vi "USRP oneTx one Rx.vi"() -> ()   [LabVIEW 2021]
uses:
  <vilib>/addons/Modulation/Analog/controls/Complex Data Waveform.ctl
  <vilib>/measure/maspectr.llb/Power Spectrum and PSD Export Mode.ctl
  system stop.vi
  <vilib>/measure/matone.llb/Extract Single Tone Information 1 Chan (CDB).vi
  <vilib>/measure/maspectr.llb/FFT Power Spectrum and PSD for 1 Chan (CDB).vi
  <instrlib>/niUSRP/niUSRP Fetch Rx Data (CDB Cluster).vi
  <instrlib>/niUSRP/niUSRP Write Tx Data (CDB Cluster).vi
  <vilib>/addons/Modulation/niAMT.lvlib
  <vilib>/measure/NI_MAPro.lvlib
  <vilib>/Analysis/NI_AALPro.lvlib
panel:
  in  "Tab Control":T1(tab)
  in  "IQ rate Tx":dbl=100000.0 format="%#_6p"
  in  "carrier frequency Tx":dbl=100000.0 format="%#_6p"
  in  "Tx Gain":dbl format="%#_6f"
  in  "Tx IP":refnum<k15>
  out "coerced IQ rate Tx":dbl=100000.0 format="%#_6p"
  out "coerced carrier frequency Tx":dbl=100000.0 format="%#_6p"
  in  "Rx IP":refnum<k15>
  in  "Rx gain":dbl format="%#_6f"
  in  "Frequency":dbl format="%#_13g"
  in  "Duration":dbl format="%#_13g"
  out "coerced IQ rate Rx":dbl=100000.0 format="%#_6p"
  out "coerced carrier frequency Rx":dbl=100000.0 format="%#_6p"
  in  "number of samples":i64=100000
  out "Waveform Graph":dbl[](graph)
  out "Received Waveform Graph":cluster{"f0":dbl, "df":dbl, "magnitude":dbl[]}(graph)
  out "detected frequency":dbl format="%.2p"
  out "detected Amplitude":dbl format="%.2p"
  out "Threshold indices":i32[](array[numeric])
  out "Threshold count":i32
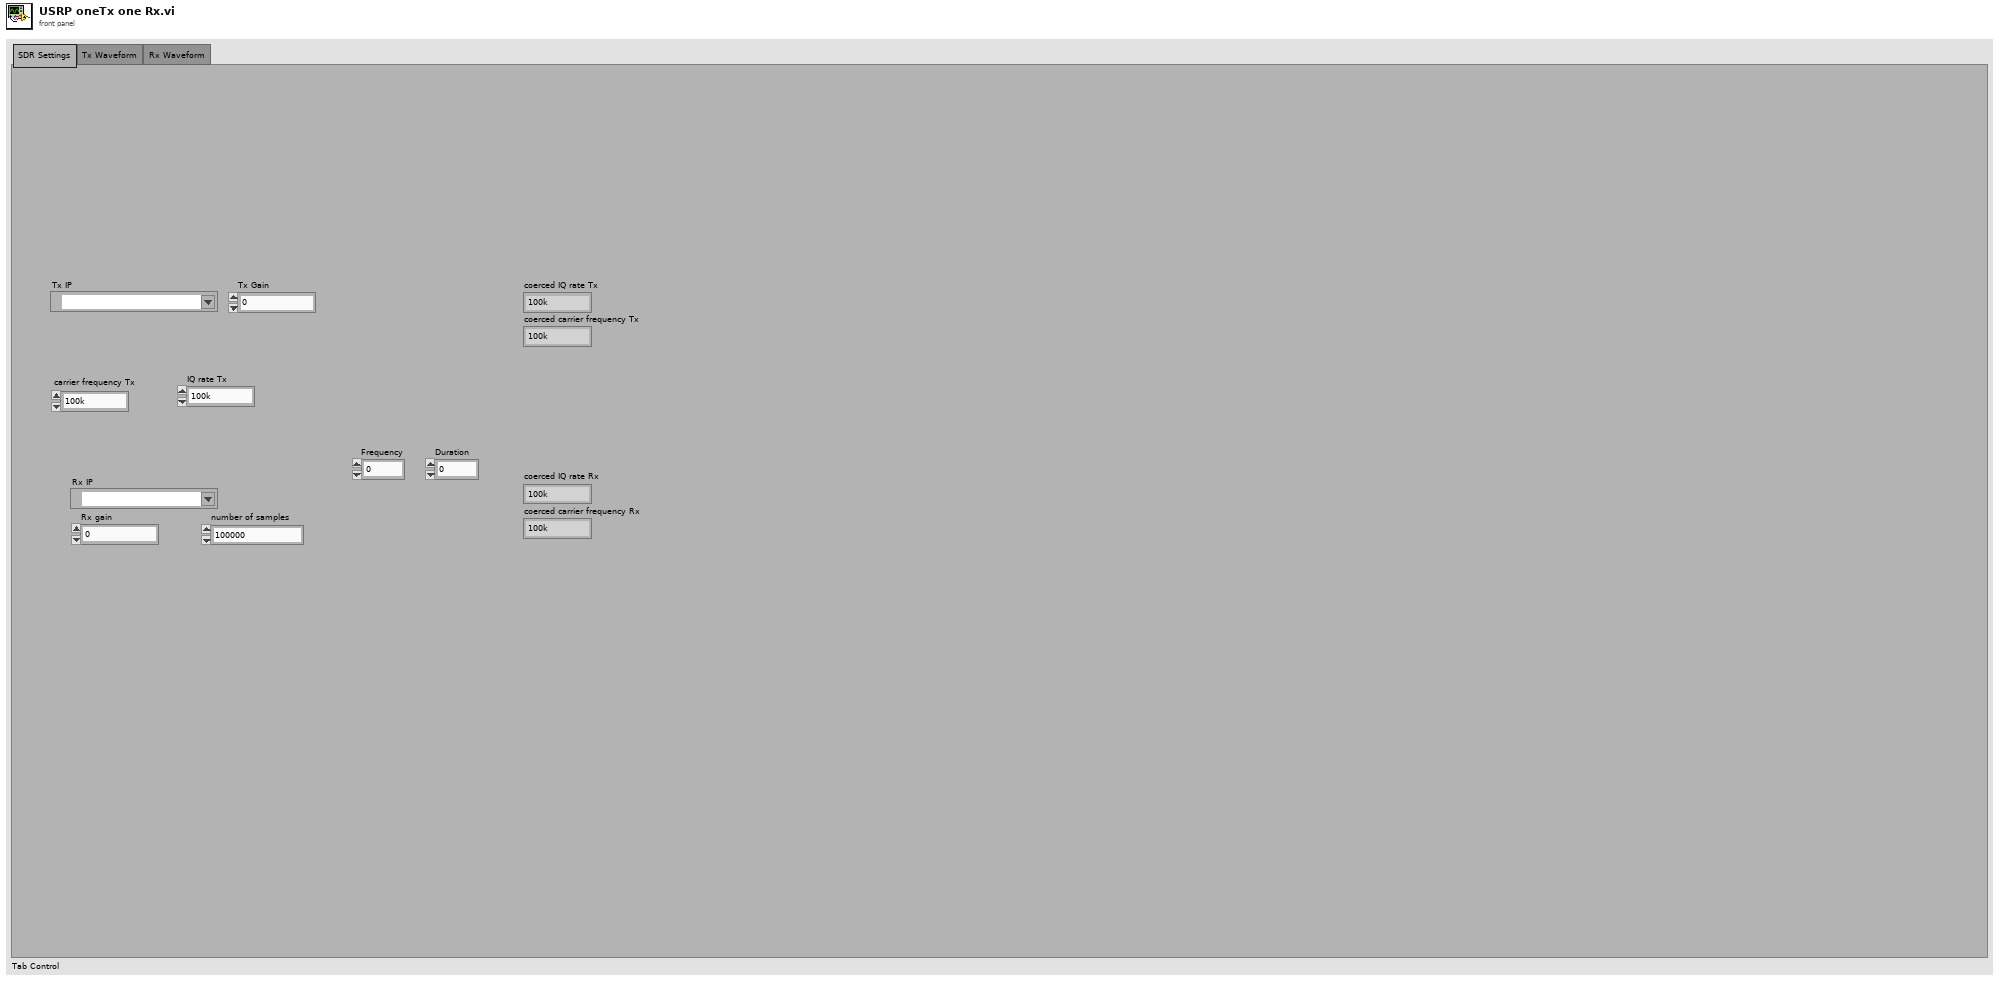
[diagram p1: front panel]
types:
  T1 = enum32{"SDR Settings", "Tx Waveform", "Rx Waveform"}
  T2 = typedef "niAMT.lvlib/Complex Data Waveform.ctl" = cluster{"t0":dbl, "dt":dbl, "Y":cdb[]}
  T3 = typedef "NI_MAPro.lvlib/Power Spectrum and PSD Export Mode.ctl" = u16
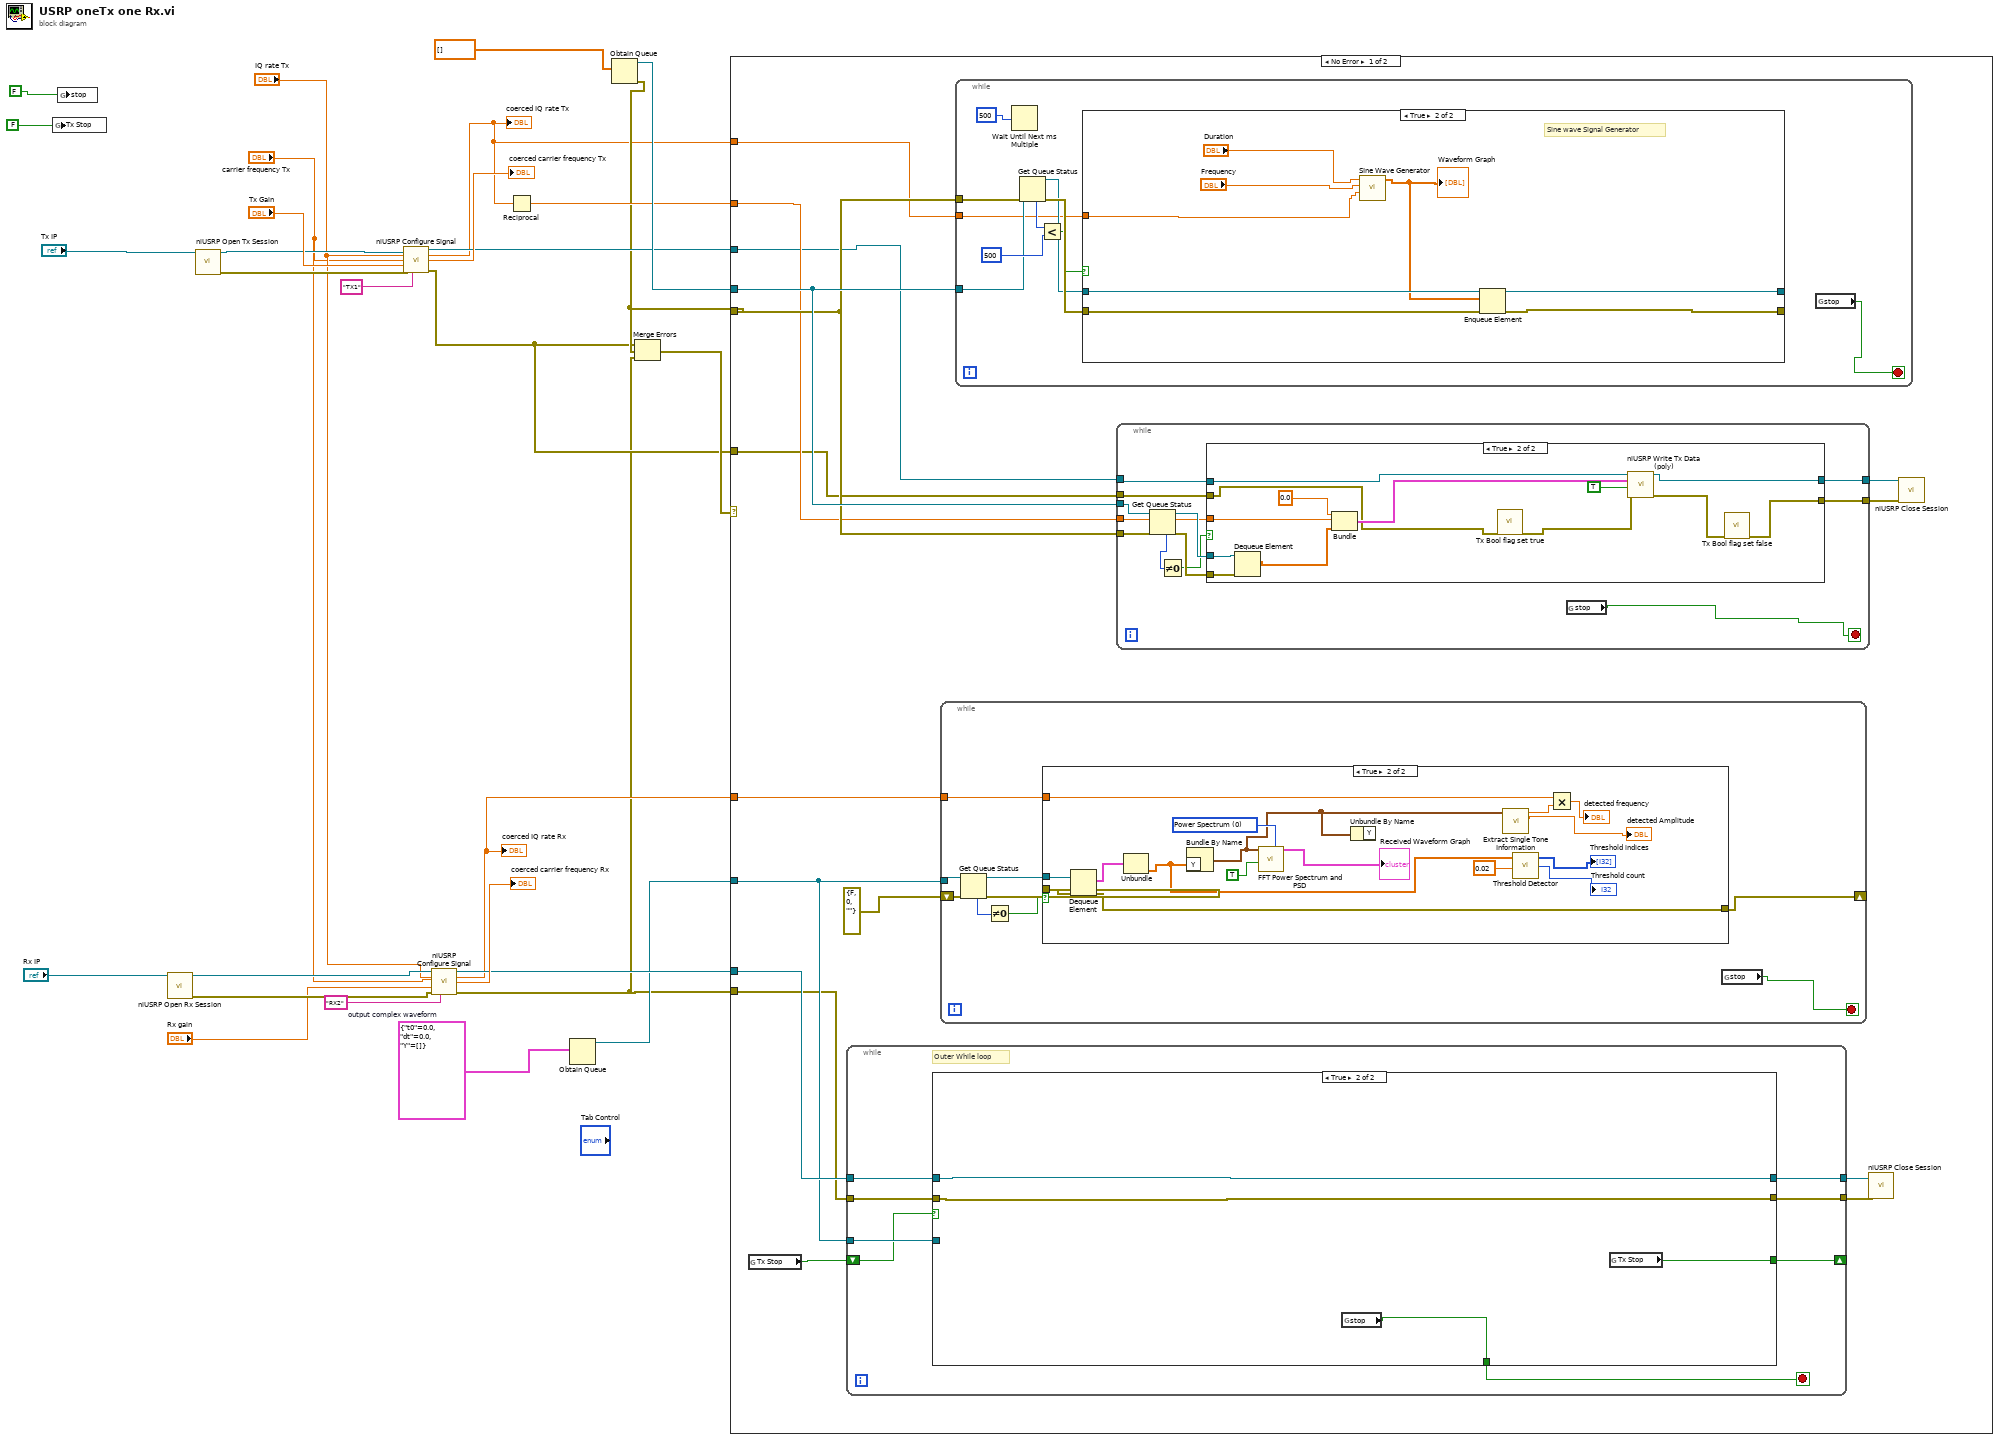
[diagram p0: block diagram]
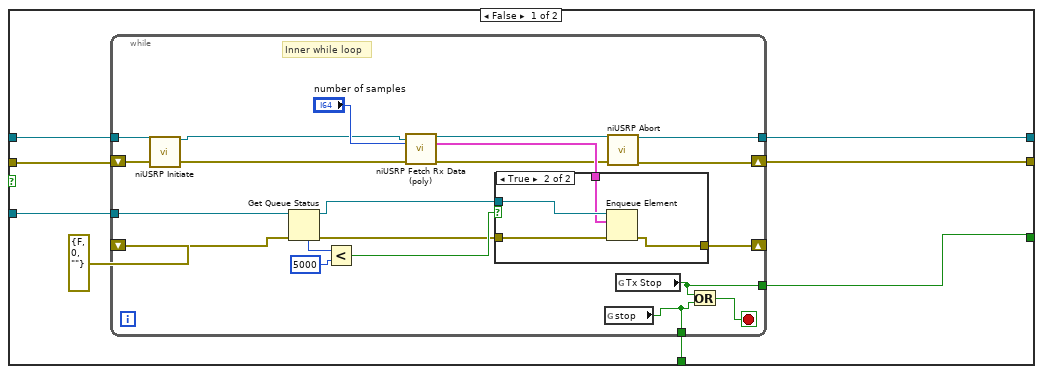
[diagram p3: hidden frame]
diagram:
  w6 = T2 {"t0"=0.0, "dt"=0.0, "Y"=[]}  # output complex waveform
  n1 = global write "system stop.vi" "Tx Stop"(FALSE) -> ()
  n2 = global write "system stop.vi" "stop"(FALSE) -> ()
  n3 = call <instrlib>:"niUSRP Open Rx Session.vi"("device names"="Rx IP") -> ("session handle out"=w13:refnum<k15>, "error out"=w12:errorcluster)  [unwired: 13 in]
  n4 = call <instrlib>:"niUSRP Open Tx Session.vi"("device names"="Tx IP") -> ("session handle out"=w27:refnum<k15>, "error out"=w26:errorcluster)  [unwired: 13 in]
  n5 = call <instrlib>:"niUSRP Configure Signal.vi"("session handle"=w27, "IQ rate"="IQ rate Tx", "carrier frequency"="carrier frequency Tx", "gain"="Tx Gain", "error in (no error)"=w26, "active antenna"="TX1") -> ("session handle out"=w20:refnum<k15>, "coerced IQ rate"=w17:dbl, "coerced carrier frequency"=→"coerced carrier frequency Tx":dbl, "error out"=w16:errorcluster)  [unwired: 5 in, 1 out]
  "coerced IQ rate Tx" <- w17
  n6 = call <instrlib>:"niUSRP Configure Signal.vi"("session handle"=w13, "IQ rate"="IQ rate Tx", "carrier frequency"="carrier frequency Tx", "gain"="Rx gain", "error in (no error)"=w12, "active antenna"="RX2") -> ("session handle out"=w7:refnum<k15>, "coerced IQ rate"=w4:dbl, "coerced carrier frequency"=→"coerced carrier frequency Rx":dbl, "error out"=w2:errorcluster)  [unwired: 5 in, 1 out]
  "coerced IQ rate Rx" <- w4
  n7 = Reciprocal(x=w17) -> (1/x=w19:dbl)
  n8 = Obtain Queue(element data type=w6) -> (queue out=w5:refnum<queue>)  [unwired: 4 in, 2 out]
  n9 = Obtain Queue(element data type=dbl[] []) -> (queue out=w21:refnum<queue>, error out=w18:errorcluster)  [unwired: 4 in, 1 out]
  n10 = Merge Errors(w16, w18, w2) -> (w23:errorcluster)
  n11 = case shown="No Error" w23 {
    tunnel: w18 -> [w44 _]
    tunnel: w21 -> [w45 _]
    tunnel: w20 -> [w42 _]
    tunnel: w19 -> [w43 _]
    tunnel: w17 -> [w41 _]
    tunnel: w16 -> [w40 _]
    tunnel: w7 -> [w38 _]
    tunnel: w5 -> [w37 _]
    tunnel: w4 -> [w36 _]
    tunnel: w2 -> [w35 _]
    frame No Error {
      n12 = global read "system stop.vi" "Tx Stop"() -> (w30:bool)
      n13 = while {
        tunnel: w38 -> [w73]
        tunnel: w37 -> [w72]
        tunnel: w35 -> [w70]
        tunnel: [w69] -> w32
        tunnel: [w68] -> w31
        shift-right: [w66] -> _
        shift-left: w30 -> [w67]
        stop <- w71 stop-if-true
        # "Outer While loop"
        n14 = case shown="True" w67 {
          tunnel: w73 -> [w78 w109]
          tunnel: w72 -> [w81 _]
          tunnel: [w79 w110] -> w71
          tunnel: w70 -> [w77 w108]
          tunnel: [w76 w109] -> w69
          tunnel: [w75 w108] -> w68
          tunnel: [w74 w107] -> w66
          frame False {
            n15 = while {
              tunnel: w81 -> [w101]
              shift-right: [w83] -> w75
              shift-left: w77 -> [w100]
              shift-right: [w99] -> _
              shift-left: errorcluster {"status"=FALSE, "code"=0, "source"=""} ("error in (no error)") -> [w98]
              tunnel: [w85] -> w79
              tunnel: w78 -> [w89]
              tunnel: [w84] -> w76
              tunnel: [w82] -> w74
              stop <- w90 stop-if-true
              # "Inner while loop"
              n16 = call <instrlib>:"niUSRP Initiate.vi"("session handle"=w89) -> ("session handle out"=w88:refnum<k15>)  [unwired: 13 in, 1 out]
              n17 = Get Queue Status(queue=w101, error in (no error)=w98) -> (queue out=w93:refnum<queue>, error out=w94:errorcluster, # elements in queue=w97:i32)  [unwired: 1 in, 5 out]
              n18 = Less?(x=w97, y=5000) -> (x < y?=w95:bool)
              n19 = call-poly <instrlib>:"niUSRP Fetch Rx Data (poly).vi"("session handle"=w88, "number of samples"="number of samples", "error in (no error)"=w100) -> ("session handle out"=w87:refnum<k15>, "data"=w91:cluster{"t0":dbl, "dt":dbl, "Y":cdb[]}, "error out"=w86:errorcluster)  [unwired: 9 in, 1 out]
              n20 = case shown="True" w95 {
                tunnel: w94 -> [w102 w106]
                tunnel: w93 -> [_ w105]
                tunnel: w91 -> [_ w104]
                tunnel: [w102 w103] -> w99
                frame False {
                }
                frame True {
                  n21 = Enqueue Element(queue=w105, element=w104, error in (no error)=w106) -> (error out=w103:errorcluster)  [unwired: 1 in, 2 out]
                }
              }
              n22 = global read "system stop.vi" "stop"() -> (w85:bool)
              n23 = call <instrlib>:"niUSRP Abort.vi"("session handle"=w87, "error in (no error)"=w86) -> ("session handle out"=w84:refnum<k15>, "error out"=w83:errorcluster)  [unwired: 12 in]
              n24 = global read "system stop.vi" "Tx Stop"() -> (w82:bool)
              n25 = Or(x=w82, y=w85) -> (x .or. y?=w90:bool)
            }
          }
          frame True {
            n26 = global read "system stop.vi" "stop"() -> (w110:bool)
            n27 = global read "system stop.vi" "Tx Stop"() -> (w107:bool)
          }
        }
      }
      n28 = while {
        tunnel: w37 -> [w116]
        shift-right: [w113] -> _
        shift-left: errorcluster {"status"=FALSE, "code"=0, "source"=""} ("error in (no error)") -> [w115]
        tunnel: w36 -> [w112]
        stop <- w111 stop-if-true
        n29 = Get Queue Status(queue=w116, error in (no error)=w115) -> (queue out=w118:refnum<queue>, error out=w117:errorcluster, # elements in queue=w119:i32)  [unwired: 1 in, 5 out]
        n30 = Not Equal To 0?(x=w119) -> (x != 0?=w114:bool)
        n31 = case shown="True" w114 {
          tunnel: w118 -> [_ w136]
          tunnel: w117 -> [w120 w125]
          tunnel: [w120 w122] -> w113
          tunnel: w112 -> [_ w121]
          frame False {
          }
          frame True {
            w133 = T3 0 items=["Power Spectrum", "Power Spectral Density"] ("export mode")
            n32 = Dequeue Element(queue=w136, error in (no error)=w125) -> (element=w124:T2, error out=w122:errorcluster)  [unwired: 1 in, 2 out]
            n33 = Unbundle(w124) -> ("Y"=w123:cdb[])  [unwired: 2 out]
            n34 = Bundle By Name("Y"=w123) -> (w129:waveform(cdb))  [unwired: 1 in]
            n35 = call-poly <vilib>:"FFT Power Spectrum and PSD.vi"("export mode"=w133, "dB On (F)"=TRUE, "time signal"=w129) -> ("Power Spectrum / PSD"=→"Received Waveform Graph":cluster{"f0":dbl, "df":dbl, "magnitude":dbl[]})  [unwired: 5 in, 3 out]
            n36 = Unbundle By Name(w129) -> ()  [unwired: 1 out]
            n37 = call-poly <vilib>:"Extract Single Tone Information.vi"("time signal in"=w129) -> ("detected amplitude"=→"detected Amplitude":dbl, "detected frequency"=w131:dbl)  [unwired: 5 in, 4 out]
            n38 = call <vilib>:"Threshold Detector.vi"("threshold"=0.02, "X"=w123) -> ("count"=→"Threshold count":i32, "Indices"=→"Threshold indices":i32[])  [unwired: 1 in, 1 out]
            n39 = Multiply(x=w121, y=w131) -> (x*y=→"detected frequency":dbl)
          }
        }
        n40 = global read "system stop.vi" "stop"() -> (w111:bool)
      }
      n41 = while {
        tunnel: w45 -> [w50]
        tunnel: w44 -> [w49]
        tunnel: w41 -> [w48]
        stop <- w46 stop-if-true
        n42 = Wait Until Next ms Multiple(millisecond multiple=500) -> ()  [unwired: 1 out]
        n43 = Get Queue Status(queue=w50, error in (no error)=w49) -> (queue out=w52:refnum<queue>, error out=w53:errorcluster, # elements in queue=w55:i32)  [unwired: 1 in, 5 out]
        n44 = Less?(x=w55, y=500) -> (x < y?=w51:bool)
        n45 = case shown="True" w51 {
          tunnel: w53 -> [w56 w65]
          tunnel: w52 -> [w57 w64]
          tunnel: [w57 w63] -> _
          tunnel: [w56 w62] -> _
          tunnel: w48 -> [_ w59]
          frame False {
          }
          frame True {
            # "Sine wave Signal Generator"
            n46 = call "SIne Wave Generator.vi"("Sampling rate"=w59, "Frequency"="Frequency", "Duration"="Duration") -> ("Array"=w58:dbl[])  [unwired: 7 in, 1 out]
            "Waveform Graph" <- w58
            n47 = Enqueue Element(queue=w64, element=w58, error in (no error)=w65) -> (queue out=w63:refnum<queue>, error out=w62:errorcluster)  [unwired: 1 in, 1 out]
          }
        }
        n48 = global read "system stop.vi" "stop"() -> (w46:bool)
      }
      n49 = while {
        tunnel: w45 -> [w148]
        tunnel: w44 -> [w145]
        tunnel: w43 -> [w144]
        tunnel: w42 -> [w142]
        tunnel: w40 -> [w140]
        tunnel: [w138] -> w34
        tunnel: [w137] -> w33
        stop <- w139 stop-if-true
        n50 = Get Queue Status(queue=w148, error in (no error)=w145) -> (queue out=w147:refnum<queue>, error out=w146:errorcluster, # elements in queue=w143:i32)  [unwired: 1 in, 5 out]
        n51 = Not Equal To 0?(x=w143) -> (x != 0?=w141:bool)
        n52 = case shown="True" w141 {
          tunnel: w147 -> [_ w163]
          tunnel: w146 -> [_ w162]
          tunnel: w144 -> [_ w161]
          tunnel: w142 -> [w150 w159]
          tunnel: w140 -> [w149 w152]
          tunnel: [w150 w155] -> w138
          tunnel: [w149 w153] -> w137
          frame False {
          }
          frame True {
            n53 = Dequeue Element(queue=w163, error in (no error)=w162) -> (element=w158:dbl[])  [unwired: 1 in, 3 out]
            n54 = Bundle(0.0, w161, w158) -> (w160:cluster{dbl, dbl, dbl[]})  [unwired: 1 in]
            n55 = call "Tx Bool flag set true.vi"("error in (no error)"=w152) -> ("error out"=w151:errorcluster)  [unwired: 9 in]
            n56 = call-poly <instrlib>:"niUSRP Write Tx Data (poly).vi"("session handle"=w159, "data"=w160, "end of data?"=TRUE, "error in (no error)"=w151) -> ("session handle out"=w155:refnum<k15>, "error out"=w154:errorcluster)  [unwired: 10 in]
            n57 = call "Tx Bool flag set false.vi"("error in (no error)"=w154) -> ("error out"=w153:errorcluster)  [unwired: 9 in]
          }
        }
        n58 = global read "system stop.vi" "stop"() -> (w139:bool)
      }
      n59 = call <instrlib>:"niUSRP Close Session.vi"("session handle"=w32, "error in (no error)"=w31) -> ()  [unwired: 13 in, 1 out]
      n60 = call <instrlib>:"niUSRP Close Session.vi"("session handle"=w34, "error in (no error)"=w33) -> ()  [unwired: 13 in, 1 out]
    }
    frame Error {
    }
  }
